vi "Initialize.vi"(7 "Channel Name":string="Setpoint.ch%d.SP", 8 "error in":errorcluster, 9 "Number of Channels":u32=1, 10 "Instance Name":string, 11 "Error in":refnum<class "Error.lvclass">) -> (0 "error out":errorcluster, 2 "Channel":T1[](array[typedef]), 3 "Error out":refnum<class "Error.lvclass">)   [LabVIEW 2023, in "Error.lvclass"]
uses:
  Error.lvclass
  Utilities/Channel.ctl
  Error.lvclass/Error.ctl
  <vilib>/ADAS Replay HIL/Channels/Tag Wrapper/Polymorphic/Open Producer Tag (I32).vi
  <vilib>/ADAS Replay HIL/Channels/Tag Wrapper/Polymorphic/Set Default Value (I32).vi
  <vilib>/ADAS Replay HIL/Channels/Tag Wrapper/Polymorphic/Open Consumer Tag (Boolean).vi
  <vilib>/ADAS Replay HIL/Channels/Tag Wrapper/Polymorphic/Set Default Value (Boolean).vi
  <vilib>/ADAS Replay HIL/Channels/Tag Wrapper/Polymorphic/Open Producer Tag (I32).vi/45cd6eaa-a1ce-41a4-8aba-62a49d103d7e.vi
  <vilib>/ADAS Replay HIL/Channels/Tag Wrapper/Polymorphic/Set Default Value (I32).vi/228e99de-6fcf-414d-86fc-dc277c7b351f.vi
  <vilib>/ADAS Replay HIL/Channels/Tag Wrapper/Polymorphic/Open Consumer Tag (Boolean).vi/bacb721e-673a-491a-accd-959f2e1f334e.vi
  <vilib>/ADAS Replay HIL/Channels/Tag Wrapper/Polymorphic/Set Default Value (Boolean).vi/228e99de-6fcf-414d-86fc-dc277c7b351f.vi
  <vilib>/ADAS Replay HIL/Channels/Tag Wrapper/Polymorphic/Open Producer Tag (I32).vi/45cd6eaa-a1ce-41a4-8aba-62a49d103d7e.vi/c28b0ead-42ad-4072-80a2-aca7f2bd7ce3.vi
  <vilib>/ADAS Replay HIL/Channels/Tag Wrapper/Polymorphic/Set Default Value (I32).vi/228e99de-6fcf-414d-86fc-dc277c7b351f.vi/4bc1c15b-36ab-481f-b8dd-c64075ce723a.vi
  <vilib>/ADAS Replay HIL/Channels/Tag Wrapper/Polymorphic/Open Consumer Tag (Boolean).vi/bacb721e-673a-491a-accd-959f2e1f334e.vi/c28b0ead-42ad-4072-80a2-aca7f2bd7ce3.vi
  <vilib>/ADAS Replay HIL/Channels/Tag Wrapper/Polymorphic/Set Default Value (Boolean).vi/228e99de-6fcf-414d-86fc-dc277c7b351f.vi/4bc1c15b-36ab-481f-b8dd-c64075ce723a.vi
  <vilib>/ADAS Replay HIL/AdasHilServices/AdasHilServices Fill In Error Info Ex.vi
  Utilities/Utilities.lvlib
  adas-replay-hil-internal/source/Channels/Tag Wrapper/Tag Wrapper.lvlib
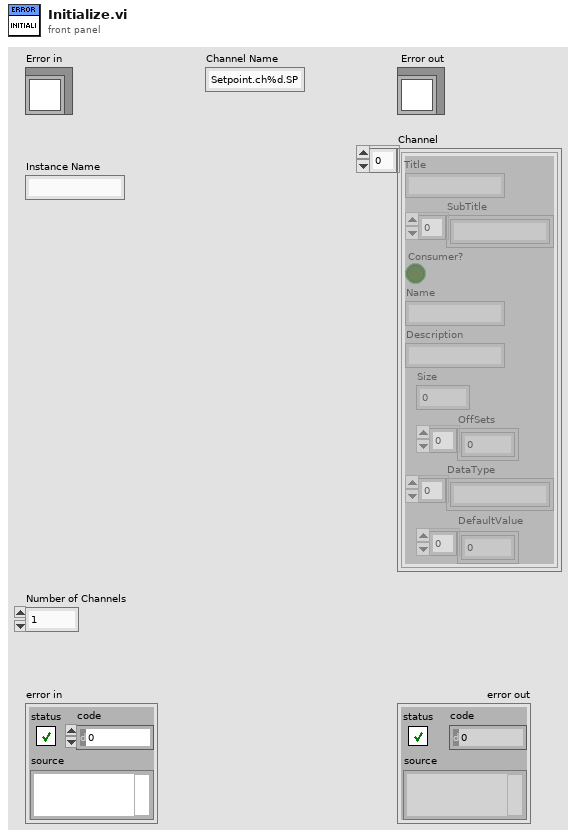
[diagram p1: front panel]
types:
  T1 = typedef "Utilities.lvlib/Channel.ctl" = cluster{"Title":string, "SubTitle":string[], "Consumer?":bool, "Name":string, "Description":string, "Size":i32, "OffSets":i32[], "DataType":string[], "DefaultValue":dbl[]}
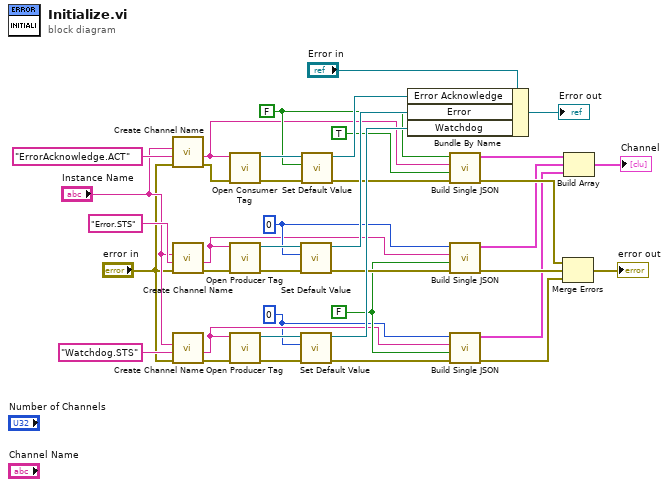
[diagram p0: block diagram]
diagram:
  w9 = FALSE ("Consumer?")
  w5 = 0 ("Default Value")
  w11 = 0 ("Default Value")
  w18 = FALSE ("Default Value")
  n1 = call "Create Channel Name.vi"("error in"="error in", "Channel Name"="ErrorAcknowledge.ACT" ("ChannelName"), "Plugin Name"="Instance Name") -> ("error out"=w38:errorcluster, "Data Channel Name"=w15:string)  [unwired: 7 in]
  n2 = call "Create Channel Name.vi"("error in"="error in", "Channel Name"="Error.STS" ("ChannelName"), "Plugin Name"="Instance Name") -> ("error out"=w34:errorcluster, "Data Channel Name"=w10:string)  [unwired: 7 in]
  n3 = call "Create Channel Name.vi"("error in"="error in", "Channel Name"="Watchdog.STS" ("ChannelName"), "Plugin Name"="Instance Name") -> ("error out"=w31:errorcluster, "Data Channel Name"=w6:string)  [unwired: 7 in]
  n4 = call-poly <vilib>:"Open Consumer Tag.vi"("error in"=w38, "Channel Name"=w15) -> ("error out"=w37:errorcluster, "ADAS HIL Channel"=w36:refnum<k21>)  [unwired: 8 in]
  n5 = call-poly <vilib>:"Open Producer Tag.vi"("error in"=w34, "Channel Name"=w10) -> ("error out"=w33:errorcluster, "ADAS HIL Channel"=w35:refnum<k21>)  [unwired: 8 in]
  n6 = call-poly <vilib>:"Open Producer Tag.vi"("error in"=w31, "Channel Name"=w6) -> ("error out"=w30:errorcluster, "ADAS HIL Channel"=w32:refnum<k21>)  [unwired: 8 in]
  n7 = call-poly <vilib>:"Set Default Value.vi"("error in"=w33, "Default Value"=w11, "ADAS HIL Channel in"=w35) -> ("error out"=w13:errorcluster, "ADAS HIL Channel out"=w23:refnum<k21>)  [unwired: 7 in]
  n8 = call-poly <vilib>:"Set Default Value.vi"("error in"=w30, "Default Value"=w5, "ADAS HIL Channel in"=w32) -> ("error out"=w8:errorcluster, "ADAS HIL Channel out"=w24:refnum<k21>)  [unwired: 7 in]
  n9 = call-poly <vilib>:"Set Default Value.vi"("error in"=w37, "Default Value"=w18, "ADAS HIL Channel in"=w36) -> ("error out"=w17:errorcluster, "ADAS HIL Channel out"=w25:refnum<k21>)  [unwired: 7 in]
  n10 = Bundle By Name(cluster="Error in", "Error Acknowledge"=w25, "Error"=w23, "Watchdog"=w24) -> (→"Error out":refnum<class "Error.lvclass">)
  n11 = call "Build Single JSON.vi"("error in"=w17, "Consumer?"=TRUE, "ChannelName"=w15, "Single"=w18) -> ("error out"=w16:errorcluster, "Channel"=w4:T1)  [unwired: 6 in]
  n12 = call "Build Single JSON.vi"("error in"=w13, "Consumer?"=w9, "ChannelName"=w10, "Single"=w11) -> ("error out"=w12:errorcluster, "Channel"=w3:T1)  [unwired: 6 in]
  n13 = call "Build Single JSON.vi"("error in"=w8, "Consumer?"=w9, "ChannelName"=w6, "Single"=w5) -> ("error out"=w7:errorcluster, "Channel"=w2:T1)  [unwired: 6 in]
  n14 = Merge Errors(w16, w12, w7) -> (→"error out":errorcluster)
  n15 = Build Array(w4, w3, w2) -> (→"Channel":T1[])
